vi "DISP_WIND_ANN_MARK_SING_STAT.vi"(0 "VISA IN":refnum<visa-resource-name>, 1 "State":bool, 5 "error in":errorcluster, 7 "Window":i32=1) -> (14 "VISA Out":refnum<visa-resource-name>, 19 "error out":errorcluster)   [LabVIEW 2018, in "PNA-X.lvlib"]
doc: "DISPlay:WINDow<wnum>:ANNotation:MARKer:SINGle[:STATe] <bool> \n(Read-Write) Either shows marker readout of only the active trace or other traces simultaneously. \nSee other SCPI Marker commands. Learn more about Marker readout. \nParameters \n<wnum> Any existing window number. If unspecified, value is set to 1. \n<bool> ON (or 1) - Shows the readout of only the active marker for each trace. \nOFF (or 0) - Shows up to 5 marker readouts per trace, up to 20 total readouts. \nExamples DISP:WIND:ANN:MARK:SING ON \ndisplay:window:annotation:marker:single off \nQuery Syntax DISPlay:WINDow:ANNotation:MARKer:SINGle? \nReturn Type Boolean (1 = ON, 0 = OFF) \nDefault OFF"
uses:
  PNA-X.lvlib
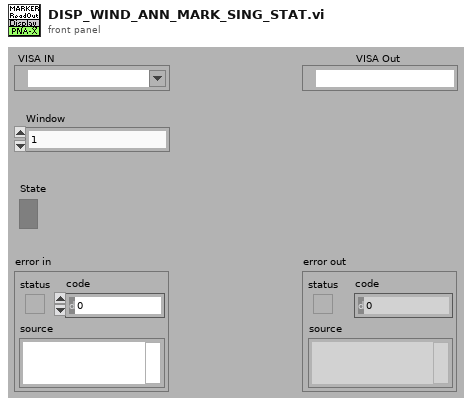
[diagram p1: front panel]
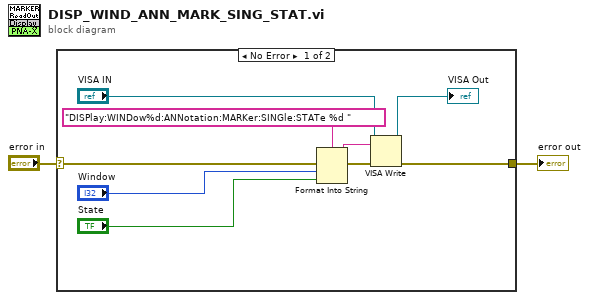
[diagram p0: block diagram]
diagram:
  n1 = case shown="No Error" "error in" {
    selector: "error in" -> [w11 w12]
    tunnel: [w6 w12] -> w1
    frame No Error {
      n2 = Format Into String(format string="DISPlay:WINDow%d:ANNotation:MARKer:SINGle:STATe %d " ("Cmdline"), error in=w11, "Window", "State") -> (resulting string=w9:string, error out=w10:errorcluster)  [unwired: 1 in]
      n3 = VISA Write(VISA resource name="VISA IN", write buffer=w9, error in (no error)=w10) -> (VISA resource name out=→"VISA Out":refnum<visa-resource-name>, error out=w6:errorcluster)  [unwired: 1 out]
    }
    frame Error {
    }
  }
  "error out" <- w1
